vi "BRig_Host__Loop_Producer__tcp_System__Data_prepareFilepaths_source.vi"(8 "input_arrFilenames":string[](array[string]), 9 "input_nFilenames":i32, 11 "input_expPrefix":string) -> (3 "output_arrPath":path[](array[path]))   [LabVIEW 2014]
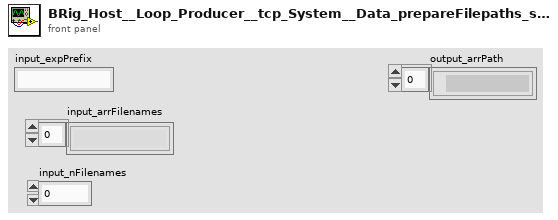
[diagram p1: front panel]
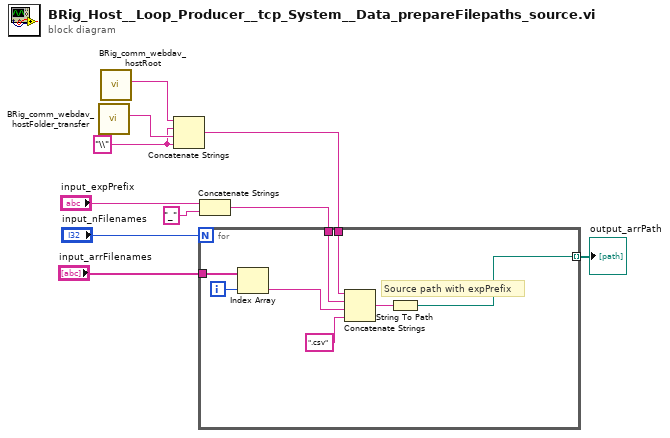
[diagram p0: block diagram]
diagram:
  w4 = "\\" ("string")
  n1 = call "BRig_comm_webdav_hostFolder_transfer.vi"() -> ("output_HostFolder"=w5:string)  [unwired: 11 in]
  n2 = call "BRig_comm_webdav_hostRoot.vi"() -> ("output_hostRoot"=w3:string)  [unwired: 11 in]
  n3 = Concatenate Strings(w3, w4, w5, w4) -> (w2:string)
  n4 = Concatenate Strings("input_expPrefix", "_" ("string")) -> (w7:string)
  n5 = for {
    N: "input_nFilenames" -> [_]
    tunnel: w7 -> [w15]
    tunnel: "input_arrFilenames" -> [w18]
    tunnel: w2 -> [w16]
    tunnel: [w14] -> w1 mode=indexing
    i -> [w17]
    # "Source path with expPrefix"
    n6 = Index Array(array=w18, index=w17) -> (element=w13:string)
    n7 = Concatenate Strings(w16, w15, w13, ".csv" ("string")) -> (w12:string)
    n8 = String To Path(string=w12) -> (path=w14:path)
  }
  "output_arrPath" <- w1
